vi "Color-Senser-Determine_Api.vi"(8 "Error In":errorcluster, 11 "HiTechnicColorSensorV2 Ref In":cluster{"I2C Ref Out":T2}) -> (0 "Error Out":errorcluster, 3 "HiTechnicColorSensorV2 Ref Out":cluster{"I2C Ref Out":T2}, 5 "對應顏色":enum16{"黃", "紅", "綠", "藍", "黑"}(ring))   [LabVIEW 2019]
uses:
  <vilib>/myRIO/Instrument Drivers/Onboard IO/I2C/typedefs/I2C Reference.ctl
  <vilib>/myRIO/Common/Instrument Driver Framework/Utilities/typedefs/myRIO Generic Hardware Reference.ctl
  <vilib>/myRIO/Common/Instrument Driver Framework/Utilities/typedefs/Hardware Version Enum.ctl
  <vilib>/myRIO/Common/Instrument Driver Framework/Utilities/typedefs/myRIO v1.0 Reference.ctl
  <vilib>/myRIO/Common/Instrument Driver Framework/Utilities/typedefs/Generic FPGA Reference.ctl
  <vilib>/myRIO/Common/Instrument Driver Framework/myRIO v1.0/I2C/typedefs/I2C Channels Enum.ctl
  <vilib>/myRIO/Instrument Drivers/Onboard IO/I2C/typedefs/I2C Configuration.ctl
  <vilib>/myRIO/Instrument Drivers/Onboard IO/I2C/typedefs/I2C Transfer Rate.ctl
  <vilib>/myRIO/Instrument Drivers/Onboard IO/DIO/typedefs/DIO Reference.ctl
  <vilib>/myRIO/Common/Instrument Driver Framework/myRIO v1.0/DIO/typedefs/DIO Channels List.ctl
  <vilib>/myRIO/Common/Instrument Driver Framework/myRIO v1.0/DIO/typedefs/DIO Channels Enum.ctl
  <vilib>/userDefined/High Color/nirio_resource_hc.ctl
  <vilib>/myRIO/Common/Instrument Driver Framework/Utilities/vis/Is FPGA Ref Available.vi
  <vilib>/myRIO/Common/Instrument Driver Framework/myRIO v1.0/DIO/vis/myRIO v1.1 Open DIO.vi
  <vilib>/myRIO/Instrument Drivers/Onboard IO/DIO/vis/Write.vi
  <vilib>/myRIO/Common/Instrument Driver Framework/Utilities/vis/Validate Channels.vi
  <vilib>/myRIO/Common/Instrument Driver Framework/myRIO v1.0/DIO/vis/myRIO v1.0 Reserve DIO.vi
  <vilib>/myRIO/Common/Instrument Driver Framework/myRIO v1.0/Resource Manager/vis/myRIO v1.0 Reserve Channel List.vi
  <vilib>/myRIO/Common/Instrument Driver Framework/myRIO v1.0/DIO/vis/myRIO v1.0 Build MUX Configuration DIO.vi
  <vilib>/myRIO/Common/Instrument Driver Framework/myRIO v1.0/Resource Manager/vis/myRIO v1.0 Reserve Channel.vi
  <vilib>/myRIO/Common/Instrument Driver Framework/myRIO v1.0/Resource Manager/vis/myRIO v1.0 Unreserve Channel.vi
  <vilib>/myRIO/Common/Instrument Driver Framework/myRIO v1.0/Resource Manager/vis/myRIO v1.0 Create Configuration List.vi
  <vilib>/myRIO/Common/Instrument Driver Framework/myRIO v1.0/Resource Manager/vis/myRIO v1.0 Build Mutex Name.vi
  Variable/Indentify-Consequent.vi
  <vilib>/Utility/VariantDataType/GetNumericInfo.vi
  <vilib>/Utility/error.llb/Error Cluster From Error Code.vi
  <vilib>/myRIO/Common/Instrument Driver Framework/myRIO v1.0/myRIO v1.1 Open.vi
  <vilib>/myRIO/Common/Instrument Driver Framework/Utilities/vis/IO Manager.vi
  <vilib>/myRIO/Common/Instrument Driver Framework/Utilities/vis/Configuration Manager.vi
  <vilib>/myRIO/Common/Instrument Driver Framework/myRIO v1.0/Resource Manager/vis/myRIO v1.0 Configure IO.vi
  <vilib>/myRIO/Common/Instrument Driver Framework/myRIO v1.0/myRIO v1.0 Close.vi
  <vilib>/myRIO/Common/Instrument Driver Framework/myRIO v1.0/DIO/vis/myRIO v1.0 Write DIO.vi
  <vilib>/myRIO/Express VI/Onboard Devices/LED/LED Express VI.xnode
  <vilib>/myRIO/Instrument Drivers/Onboard IO/DIO/vis/myRIO DIO Open.xnode
  <vilib>/myRIO/Instrument Drivers/Onboard IO/DIO/DIO.lvlib
  <vilib>/myRIO/Instrument Drivers/Onboard IO/I2C/I2C.lvlib
panel:
  out "當前顏色值":T1(array[cluster])
  out "Green or Saturation":i32
  out "Red or Hue":i32
  in  "Stop":bool
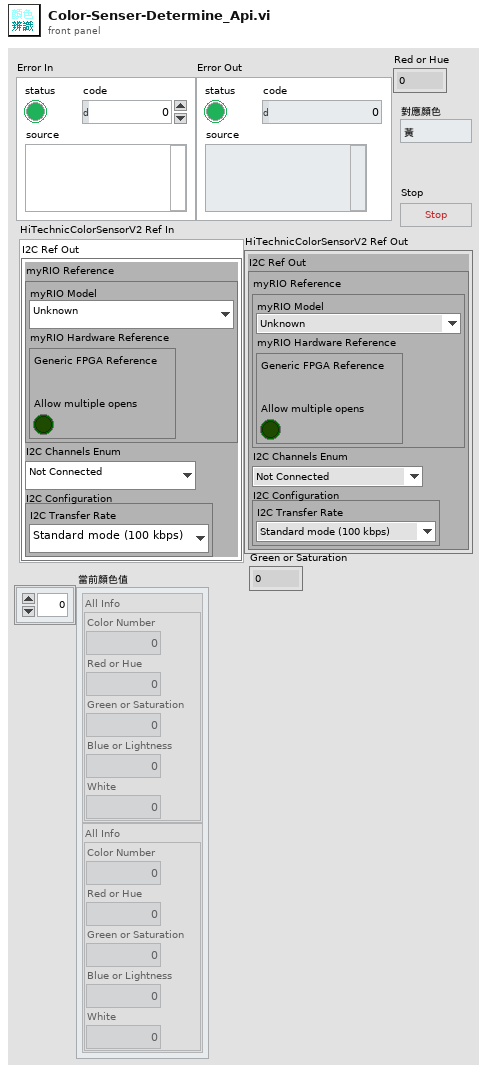
[diagram p1: front panel]
types:
  T1 = cluster{"All Info":cluster{"Color Number":i32, "Red or Hue":i32, "Green or Saturation":i32, "Blue or Lightness":i32, "White":i32}}[]
  T2 = typedef "I2C.lvlib/I2C Reference.ctl" = cluster{"myRIO Reference":T3, "I2C Channels Enum":T7, "I2C Configuration":T8}
  T3 = typedef "myRIO Generic Hardware Reference.ctl" = cluster{"myRIO Model":T4, "myRIO Hardware Reference":T5}
  T4 = typedef "Hardware Version Enum.ctl" = enum16{"Unknown", "myRIO-1900", "myRIO-1950", "roboRIO", "NI ELVIS RIO CM", "ELVIS III"}
  T5 = typedef "myRIO v1.0 Reference.ctl" = cluster{"Generic FPGA Reference":T6, "Allow multiple opens":bool}
  T6 = typedef "Generic FPGA Reference.ctl" = refnum<k20>
  T7 = typedef "I2C Channels Enum.ctl" = enum16{"Not Connected", "A/I2C", "B/I2C", "I2C/I2C"}
  T8 = typedef "I2C.lvlib/I2C Configuration.ctl" = cluster{"I2C Transfer Rate":T9}
  T9 = typedef "I2C.lvlib/I2C Transfer Rate.ctl" = enum16{"Standard mode (100 kbps)", "Fast mode (400 kbps)"}
  T10 = cluster{"All Info":cluster{"Color Number":i32, "Red or Hue":i32, "Green or Saturation":i32, "Blue or Lightness":i32, "White":i32}}
  T11 = cluster{"Color Number":i32, "Red or Hue":i32, "Green or Saturation":i32, "Blue or Lightness":i32, "White":i32}
  T12 = typedef "DIO.lvlib/DIO Reference.ctl" = cluster{"myRIO Reference":T3, "DIO Channels List":T13}
  T13 = typedef "DIO Channels List.ctl" = T14[]
  T14 = typedef "DIO Channels Enum.ctl" = enum16{"Not Connected", "C/DIO0", "C/DIO1", "C/DIO2", "C/DIO3", "C/DIO4", "C/DIO5", "C/DIO6", "C/DIO7", "A/DIO0", "A/DIO1", "A/DIO2", "A/DIO3", "A/DIO4", "A/DIO5", "A/DIO6", "A/DIO7", "A/DIO8", "A/DIO9", "A/DIO10", "A/DIO11", "A/DIO12", "A/DIO13", "A/DIO14", "A/DIO15", "A/DIO16", "A/DIO17", "A/DIO18", "A/DIO19", "B/DIO0", "B/DIO1", "B/DIO2", "B/DIO3", "B/DIO4", "B/DIO5", "B/DIO6", "B/DIO7", "B/DIO8", "B/DIO9", "B/DIO10", "B/DIO11", "B/DIO12", "B/DIO13", "B/DIO14", "B/DIO15", "B/DIO16", "B/DIO17", "B/DIO18", "B/DIO19", "LED0", "LED1", "LED2", "LED3", "Button0", "DIO/DIO0", "DIO/DIO1", "DIO/DIO2", "DIO/DIO3", "DIO/DIO4", "DIO/DIO5", "DIO/DIO6", "DIO/DIO7", "DIO/DIO8", "DIO/DIO9", "SPI/CS0", "SPI/CS1", "SPI/CS2", "SPI/CS3", "LED RADIO (Green)", "LED RADIO (Red)", "LED COMM (Green)", "LED COMM (Red)", "LED MODE (Green)", "LED MODE (Red)"}
  T15 = typedef "nirio_resource_hc.ctl" = tag
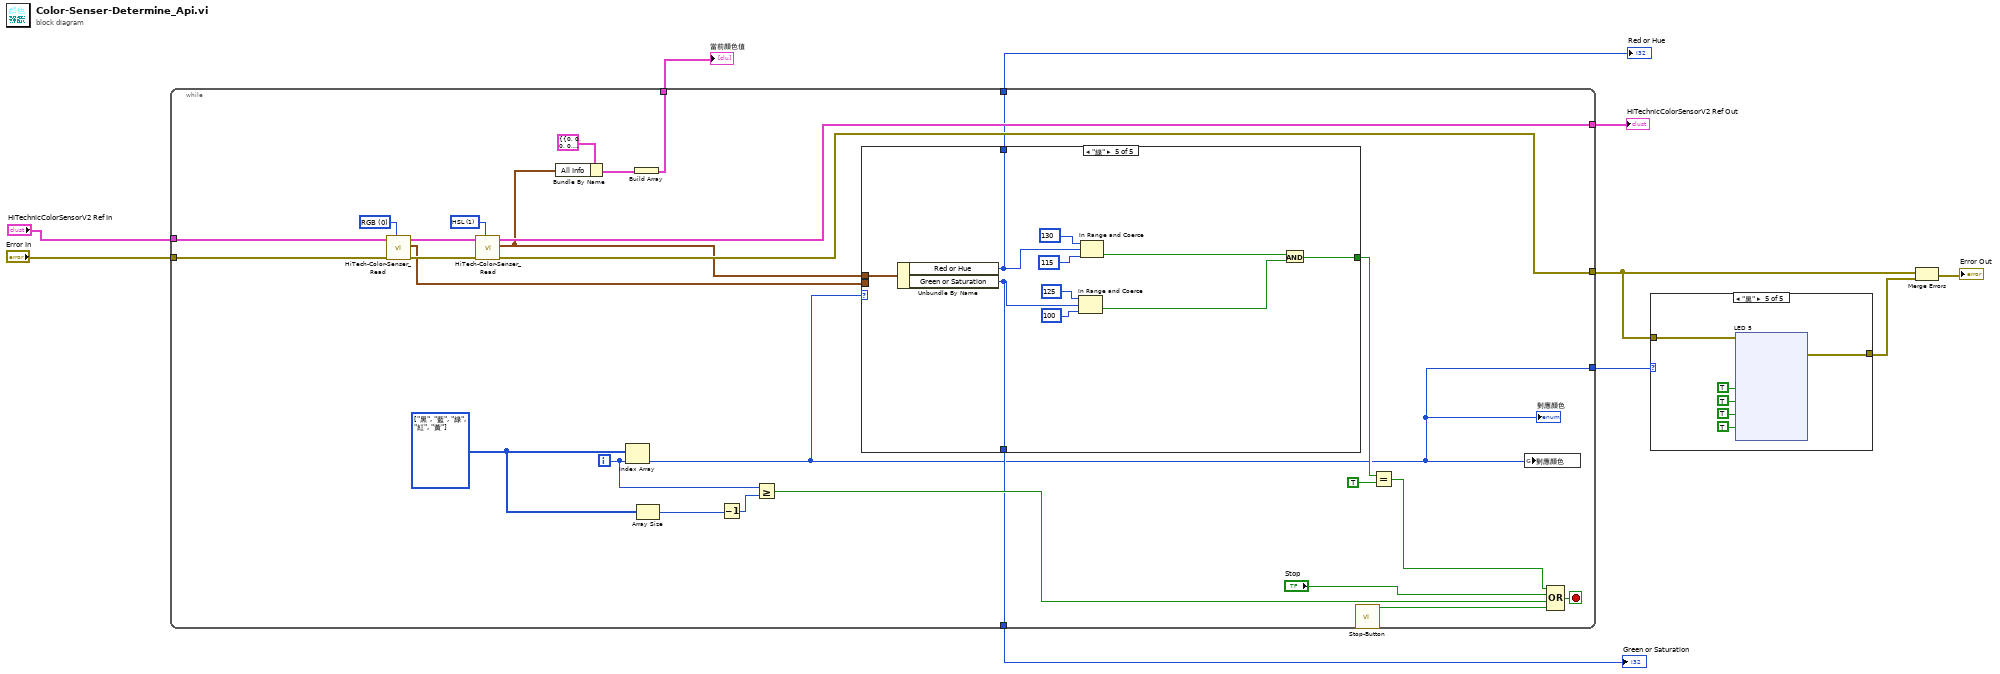
[diagram p0: block diagram]
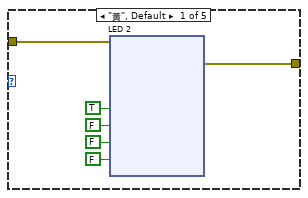
[diagram p2: hidden frame]
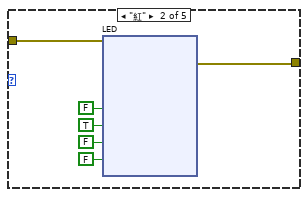
[diagram p3: hidden frame]
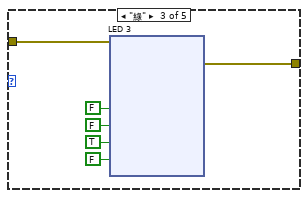
[diagram p4: hidden frame]
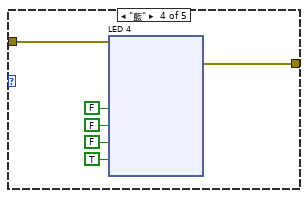
[diagram p5: hidden frame]
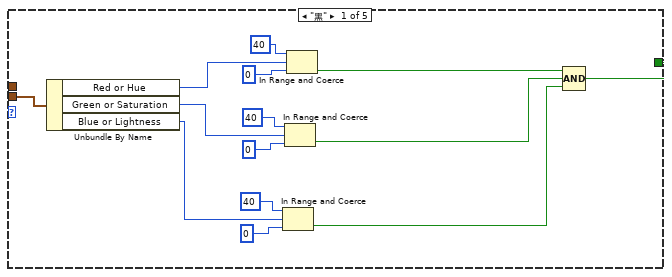
[diagram p6: hidden frame]
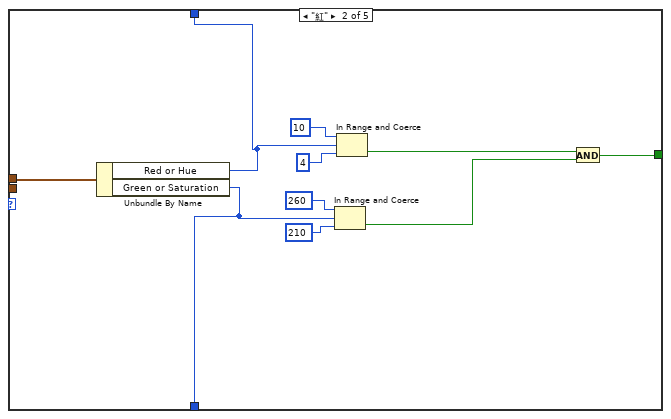
[diagram p7: hidden frame]
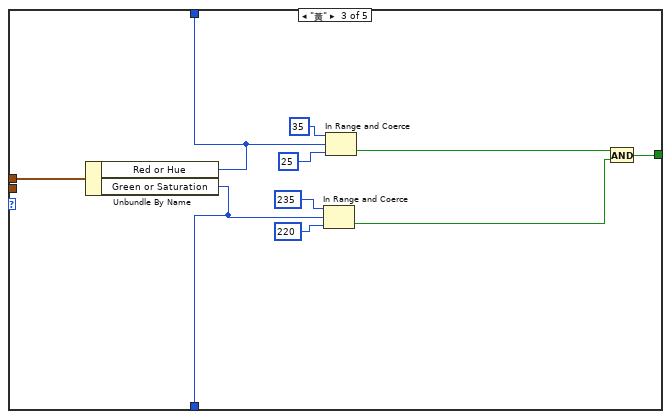
[diagram p8: hidden frame]
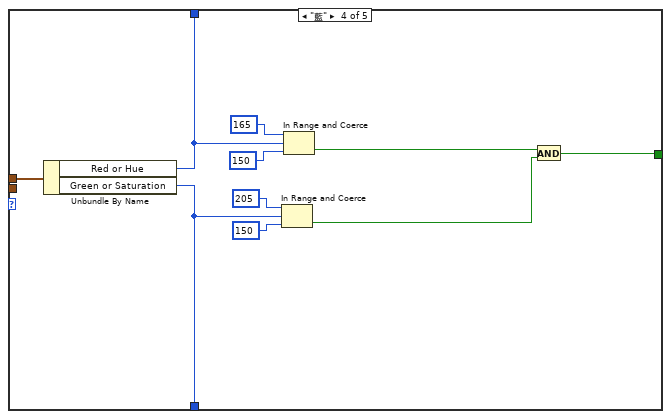
[diagram p9: hidden frame]
diagram:
  n1 = while {
    tunnel: [w33] -> w2
    tunnel: [w32] -> w10
    tunnel: "Error In" -> [w22]
    tunnel: "HiTechnicColorSensorV2 Ref In" -> [w21]
    tunnel: [w19] -> w7
    tunnel: [w18] -> w6
    tunnel: [w13] -> w5
    tunnel: [w12] -> w4
    i -> [w27]
    stop <- w28 stop-if-true
    w31 = u16 0 items=["RGB", "HSL", "HSV", "HSI", "CIE L*a*b*", "CIE XYZ"] ("Color Mode")
    w34 = enum16{"黃", "紅", "綠", "藍", "黑"}[] [enum."黑", enum."藍", enum."綠", enum."紅", enum."黃"] items=["黃", "紅", "綠", "藍", "黑"]
    w37 = u16 1 items=["RGB", "HSL", "HSV", "HSI", "CIE L*a*b*", "CIE XYZ"] ("Color Mode")
    n2 = call "HiTech-Color-Senser_Read.vi"("Color Mode"=w31, "Error In"=w22, "HiTechnicColorSensorV2 Ref In"=w21) -> ("Error Out"=w30:errorcluster, "All Info"=w16:T11, "HiTechnicColorSensorV2 Ref Out"=w29:cluster{"I2C Ref Out":T2})  [unwired: 6 in]
    n3 = call "HiTech-Color-Senser_Read.vi"("Color Mode"=w37, "Error In"=w30, "HiTechnicColorSensorV2 Ref In"=w29) -> ("Error Out"=w33:errorcluster, "All Info"=w17:T11, "HiTechnicColorSensorV2 Ref Out"=w32:cluster{"I2C Ref Out":T2})  [unwired: 6 in]
    n4 = Bundle By Name(cluster=T10 {"All Info"={"Color Number"=0, "Red or Hue"=0, "Green or Saturation"=0, "Blue or Lightness"=0, "White"=0}} ("input cluster"), "All Info"=w17) -> (w15:T10)
    n5 = Index Array(array=w34, index=w27) -> (element=w12:enum16{"黃", "紅", "綠", "藍", "黑"})
    "對應顏色" <- w12
    n6 = Build Array(w15) -> (w13:T1)
    n7 = Array Size(array=w34) -> (size(s)=w36:i32)
    n8 = Decrement(x=w36) -> (x-1=w35:i32)
    n9 = Greater Or Equal?(x=w27, y=w35) -> (x >= y?=w26:bool)
    n10 = case shown="\"綠\"" w12 {
      tunnel: w17 -> [_ w58 w67 w77 w87]
      tunnel: w16 -> [w45 _ _ _ _]
      tunnel: [w38 w54 w64 w74 w84] -> w23
      tunnel: [_ w53 w63 w72 w83] -> w19
      tunnel: [_ w52 w62 w73 w82] -> w18
      frame "黑" {
        n11 = Unbundle By Name(w45) -> ("Red or Hue"=w51:i32, "Green or Saturation"=w50:i32, "Blue or Lightness"=w42:i32)
        n12 = In Range and Coerce(upper limit=40, x=w42, lower limit=0) -> (In Range?=w39:bool)  [unwired: 1 out]
        n13 = In Range and Coerce(upper limit=40, x=w50, lower limit=0) -> (In Range?=w40:bool)  [unwired: 1 out]
        n14 = In Range and Coerce(upper limit=40, x=w51, lower limit=0) -> (In Range?=w41:bool)  [unwired: 1 out]
        n15 = Compound Arithmetic op=AND(w41, w40, w39) -> (w38:bool)
      }
      frame "紅" {
        n16 = Unbundle By Name(w58) -> ("Red or Hue"=w53:i32, "Green or Saturation"=w52:i32)
        n17 = In Range and Coerce(upper limit=260, x=w52, lower limit=210) -> (In Range?=w55:bool)  [unwired: 1 out]
        n18 = In Range and Coerce(upper limit=10, x=w53, lower limit=4) -> (In Range?=w56:bool)  [unwired: 1 out]
        n19 = And(x=w56, y=w55) -> (x .and. y?=w54:bool)
      }
      frame "黃" {
        n20 = Unbundle By Name(w67) -> ("Red or Hue"=w63:i32, "Green or Saturation"=w62:i32)
        n21 = In Range and Coerce(upper limit=235, x=w62, lower limit=220) -> (In Range?=w65:bool)  [unwired: 1 out]
        n22 = In Range and Coerce(upper limit=35, x=w63, lower limit=25) -> (In Range?=w66:bool)  [unwired: 1 out]
        n23 = And(x=w66, y=w65) -> (x .and. y?=w64:bool)
      }
      frame "藍" {
        n24 = Unbundle By Name(w77) -> ("Red or Hue"=w72:i32, "Green or Saturation"=w73:i32)
        n25 = In Range and Coerce(upper limit=205, x=w73, lower limit=150) -> (In Range?=w75:bool)  [unwired: 1 out]
        n26 = In Range and Coerce(upper limit=165, x=w72, lower limit=150) -> (In Range?=w76:bool)  [unwired: 1 out]
        n27 = And(x=w76, y=w75) -> (x .and. y?=w74:bool)
      }
      frame "綠" {
        n28 = Unbundle By Name(w87) -> ("Red or Hue"=w83:i32, "Green or Saturation"=w82:i32)
        n29 = In Range and Coerce(upper limit=125, x=w82, lower limit=100) -> (In Range?=w85:bool)  [unwired: 1 out]
        n30 = In Range and Coerce(upper limit=130, x=w83, lower limit=115) -> (In Range?=w86:bool)  [unwired: 1 out]
        n31 = And(x=w86, y=w85) -> (x .and. y?=w84:bool)
      }
    }
    n32 = call "Stop-Button.vi"() -> ("顯示按下?"=w20:bool)  [unwired: 10 in, 1 out]
    n33 = Equal?(x=w23, y=TRUE) -> (x = y?=w11:bool)
    n34 = global write "Indentify-Consequent.vi" "對應顏色"(w12) -> ()
    n35 = Compound Arithmetic op=OR(w11, "Stop", w26, w20) -> (w28:bool)
  }
  "HiTechnicColorSensorV2 Ref Out" <- w10
  "Red or Hue" <- w7
  "Green or Saturation" <- w6
  "當前顏色值" <- w5
  n36 = case shown="\"黑\"" w4 {
    tunnel: w2 -> [w93 w137 w181 w225 w269]
    tunnel: [w92 w136 w180 w224 w268] -> w1
    frame "黃", Default {
      n37 = xnode "LED 2"("LED0"=TRUE, "LED1"=FALSE, "LED2"=FALSE, "LED3"=FALSE, "error in (no error)"=w93) -> ("error out"=w92:errorcluster)
    }
    frame "紅" {
      n38 = xnode "LED"("LED0"=FALSE, "LED1"=TRUE, "LED2"=FALSE, "LED3"=FALSE, "error in (no error)"=w137) -> ("error out"=w136:errorcluster)
    }
    frame "綠" {
      n39 = xnode "LED 3"("LED0"=FALSE, "LED1"=FALSE, "LED2"=TRUE, "LED3"=FALSE, "error in (no error)"=w181) -> ("error out"=w180:errorcluster)
    }
    frame "藍" {
      n40 = xnode "LED 4"("LED0"=FALSE, "LED1"=FALSE, "LED2"=FALSE, "LED3"=TRUE, "error in (no error)"=w225) -> ("error out"=w224:errorcluster)
    }
    frame "黑" {
      n41 = xnode "LED 5"("LED0"=TRUE, "LED1"=TRUE, "LED2"=TRUE, "LED3"=TRUE, "error in (no error)"=w269) -> ("error out"=w268:errorcluster)
    }
  }
  n42 = Merge Errors(w2, w1) -> (→"Error Out":errorcluster)
